vi "ScanInfo.vi"(8 "error in (no error)":errorcluster, 11 "scan info":refnum<k24>) -> (0 "error out":errorcluster, 3 "VGS_ScanInfo out":refnum<class "VGS_ScanInfo.lvclass">)   [LabVIEW 2022 SP3, in "LV_VGS.lvlib" / "VGS_ScanInfo.lvclass"]
uses:
  VGS_ScanInfo.lvclass
  C:/Users/Andrey/Documents/GitHub/LV_VGS/vgs_project.dll
  vgs_project.dll
  VGS_ScanInfo.lvclass/VGS_ScanInfo.ctl
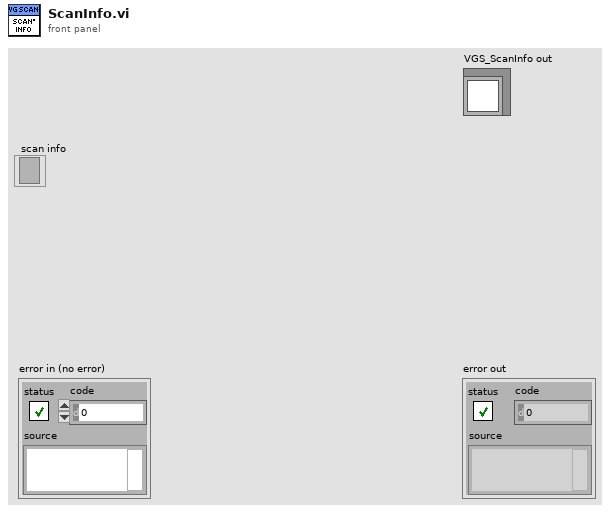
[diagram p1: front panel]
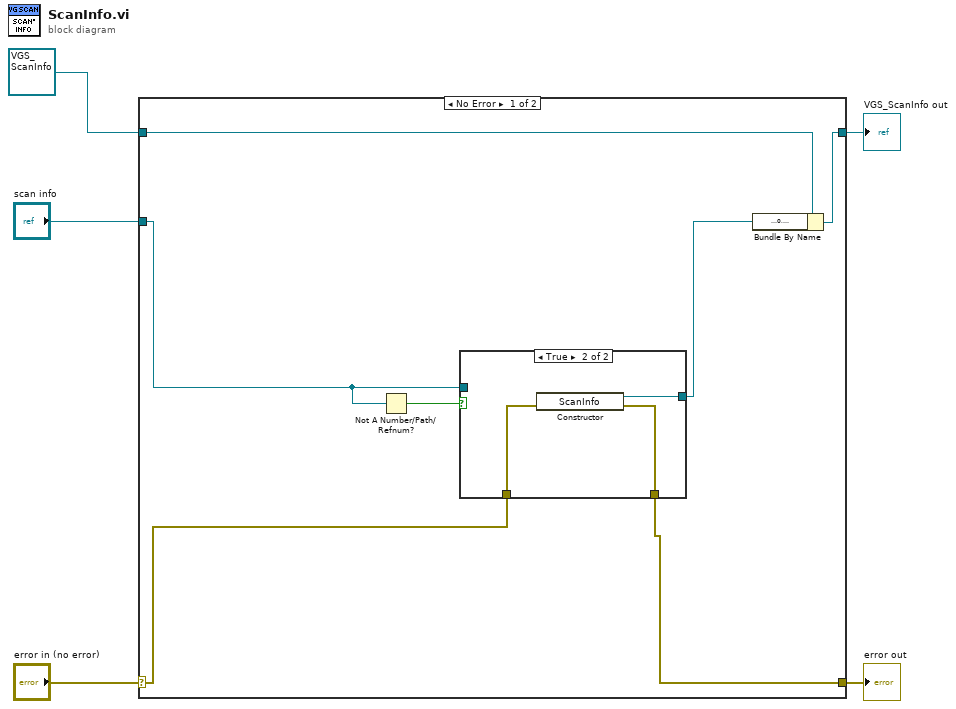
[diagram p0: block diagram]
diagram:
  n1 = case shown="No Error" "error in (no error)" {
    selector: "error in (no error)" -> [w7 w18]
    tunnel: [w6 w18] -> w4
    tunnel: [w11 w19] -> w2
    tunnel: refnum<class "VGS_ScanInfo.lvclass"> refnum ("VGS_ScanInfo in") -> [w12 w19]
    tunnel: "scan info" -> [w9 _]
    frame No Error {
      n2 = Not A Number/Path/Refnum?(number/path/refnum=w9) -> (NaN/Path/Refnum?=w10:bool)
      n3 = case shown="True" w10 {
        tunnel: [w14 w17] -> w8
        tunnel: w7 -> [w13 w16]
        tunnel: [w13 w15] -> w6
        tunnel: w9 -> [w14 _]
        frame False {
        }
        frame True {
          n4 = constructor class="ScanInfo"(error in=w16) -> (reference out=w17:refnum<k24>, error out=w15:errorcluster)  [unwired: 2 in, 1 out]
        }
      }
      n5 = Bundle By Name(cluster=w12, "scan info"=w8) -> (w11:refnum<class "VGS_ScanInfo.lvclass">)
    }
    frame Error {
    }
  }
  "error out" <- w4
  "VGS_ScanInfo out" <- w2
